vi "New Stainless Correction Pop Up.vi"(2 "New Feet\n of Stainless\n(Count)":i32) -> (0 "Feet of\nStainless to be\nUsed (Count)":i32)   [LabVIEW 2016]
doc: "This vi allows the clinician to input the starting flexion. It used in order to derive a flexion correction."
uses:
  Kpro Globals.vi
panel:
  out "Depth to Water Table":dbl=-5.0 format="%.2f"
  out "Original Feet\n of Stainless\n(Count)":i32
  in  "stop":bool
  in  "Increment Stainless":bool
  in  "Stainless OK As Is":bool
  in  "Correct Stainless":bool
  # "Please Choose \nto Correct, Increment, or to \nLeave Feet of Stainless as is"
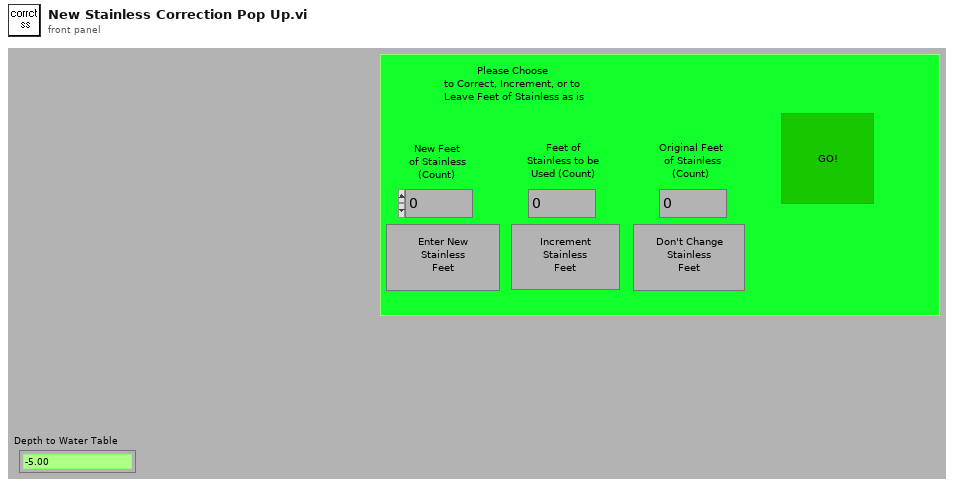
[diagram p1: front panel]
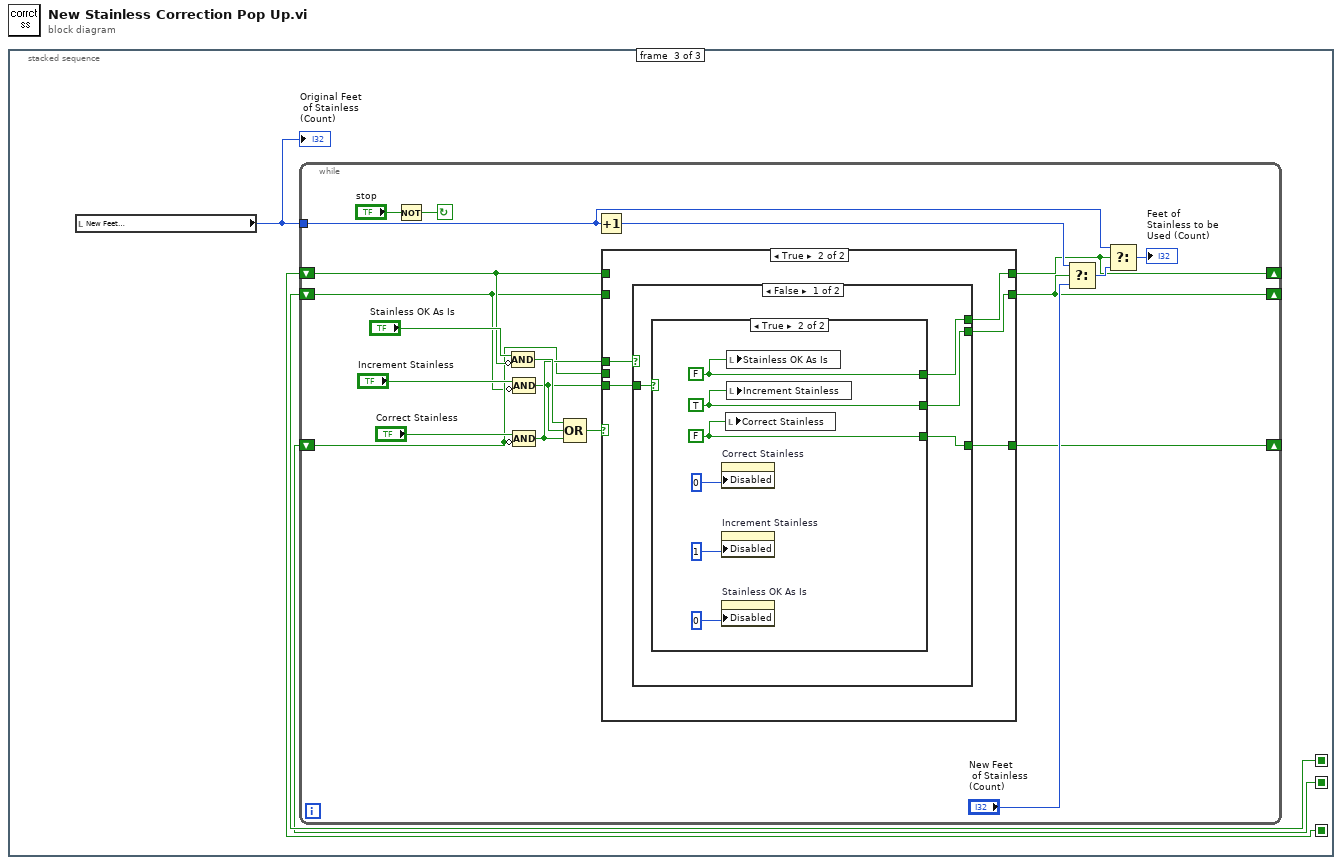
[diagram p0: block diagram]
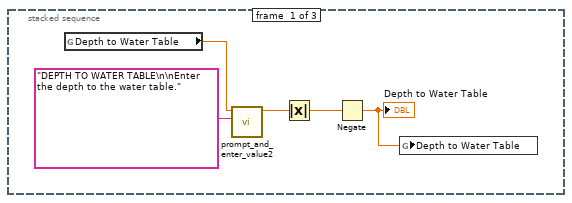
[diagram p2: hidden frame]
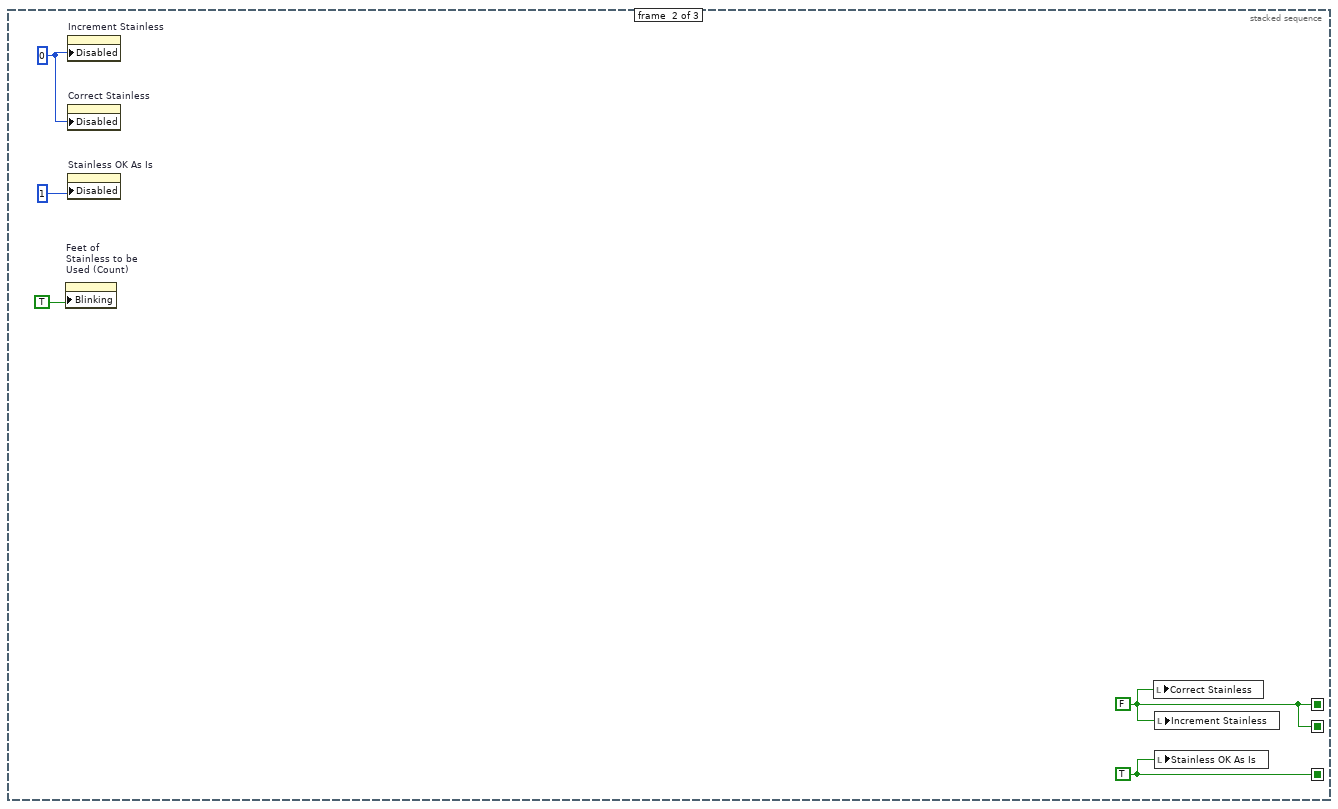
[diagram p3: hidden frame]
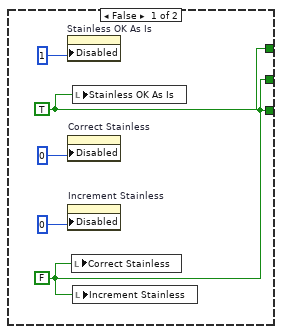
[diagram p5: hidden frame]
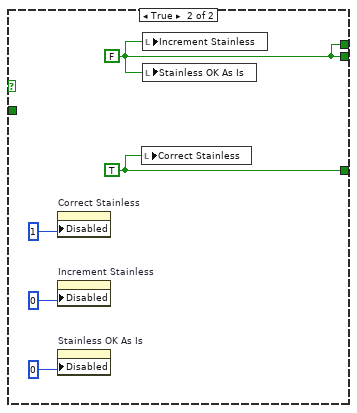
[diagram p6: hidden frame]
diagram:
  n1 = stacked-sequence {
    seq-local: [_ w9 _] -> [_ _ w12]
    seq-local: [_ w9 _] -> [_ _ w13]
    seq-local: [_ w10 _] -> [_ _ w14]
    frame #0 {
      n2 = global read "Kpro Globals.vi" "Depth to Water Table"() -> (w5:dbl)
      n3 = call "prompt_and_enter_value2.vi"("prompt_IN"="DEPTH TO WATER TABLE\n\nEnter the depth to the water table." ("prompt"), "Enter value"=w5) -> ("Numeric"=w1:dbl)  [unwired: 9 in]
      n4 = Absolute Value(x=w1) -> (abs(x)=w2:dbl)
      n5 = Negate(x=w2) -> (-x=w3:dbl)
      "Depth to Water Table" <- w3
      n6 = global write "Kpro Globals.vi" "Depth to Water Table"(w3) -> ()
    }
    frame #1 {
      w7 = 0
      w10 = TRUE
      w9 = FALSE
      n7 = property on="Feet of\nStainless to be\nUsed (Count)" class="DigNum (strict)"("Blinking"=TRUE) -> ()  [unwired: 2 in, 2 out]
      n8 = property on="Increment Stainless" class="Bool (strict)"("Disabled"=w7) -> ()  [unwired: 2 in, 2 out]
      n9 = property on="Correct Stainless" class="Bool (strict)"("Disabled"=w7) -> ()  [unwired: 2 in, 2 out]
      n10 = property on="Stainless OK As Is" class="Bool (strict)"("Disabled"=1) -> ()  [unwired: 2 in, 2 out]
      n11 = local write "Correct Stainless"(w9) -> ()
      n12 = local write "Increment Stainless"(w9) -> ()
      n13 = local write "Stainless OK As Is"(w10) -> ()
    }
    frame #2 {
      n14 = local read "New Feet\n of Stainless\n(Count)"() -> (w11:i32)
      "Original Feet\n of Stainless\n(Count)" <- w11
      n15 = while {
        tunnel: w11 -> [w16]
        shift-left: w12 -> [w18]
        shift-right: [w23] -> _
        shift-left: w13 -> [w17]
        shift-right: [w24] -> _
        shift-left: w14 -> [w19]
        shift-right: [w15] -> _
        stop <- w20 continue-if-true
        n16 = Not(x="stop") -> (.not. x?=w20:bool)
        n17 = Compound Arithmetic op=AND("Stainless OK As Is", invert w19) -> (w26:bool)
        n18 = Compound Arithmetic op=AND("Increment Stainless", invert w17) -> (w21:bool)
        n19 = Compound Arithmetic op=AND("Correct Stainless", invert w18) -> (w22:bool)
        n20 = Compound Arithmetic op=OR(w26, w21, w22) -> (w25:bool)
        n21 = Increment(x=w16) -> (x+1=w33:i32)
        n22 = case shown="True" w25 {
          tunnel: [w37 w40] -> w15
          tunnel: [w36 w39] -> w24
          tunnel: [w35 w41] -> w23
          tunnel: w22 -> [_ w42]
          tunnel: w21 -> [_ w38]
          tunnel: w19 -> [w37 _]
          tunnel: w18 -> [w35 _]
          tunnel: w17 -> [w36 _]
          frame False {
          }
          frame True {
            n23 = case shown="False" w42 {
              tunnel: [w43 w62] -> w41
              tunnel: [w45 w61] -> w40
              tunnel: [w44 w61] -> w39
              tunnel: w38 -> [w46 _]
              frame False {
                n24 = case shown="True" w46 {
                  tunnel: [w50 w55] -> w45
                  tunnel: [w51 w56] -> w44
                  tunnel: [w51 w57] -> w43
                  frame False {
                    w50 = TRUE
                    w51 = FALSE
                    n25 = property on="Stainless OK As Is" class="Bool (strict)"("Disabled"=1) -> ()  [unwired: 2 in, 2 out]
                    n26 = property on="Correct Stainless" class="Bool (strict)"("Disabled"=0) -> ()  [unwired: 2 in, 2 out]
                    n27 = property on="Increment Stainless" class="Bool (strict)"("Disabled"=0) -> ()  [unwired: 2 in, 2 out]
                    n28 = local write "Correct Stainless"(w51) -> ()
                    n29 = local write "Stainless OK As Is"(w50) -> ()
                    n30 = local write "Increment Stainless"(w51) -> ()
                  }
                  frame True {
                    w55 = FALSE
                    w56 = TRUE
                    w57 = FALSE
                    n31 = property on="Correct Stainless" class="Bool (strict)"("Disabled"=0) -> ()  [unwired: 2 in, 2 out]
                    n32 = property on="Increment Stainless" class="Bool (strict)"("Disabled"=1) -> ()  [unwired: 2 in, 2 out]
                    n33 = property on="Stainless OK As Is" class="Bool (strict)"("Disabled"=0) -> ()  [unwired: 2 in, 2 out]
                    n34 = local write "Correct Stainless"(w57) -> ()
                    n35 = local write "Stainless OK As Is"(w55) -> ()
                    n36 = local write "Increment Stainless"(w56) -> ()
                  }
                }
              }
              frame True {
                w61 = FALSE
                w62 = TRUE
                n37 = property on="Correct Stainless" class="Bool (strict)"("Disabled"=1) -> ()  [unwired: 2 in, 2 out]
                n38 = property on="Increment Stainless" class="Bool (strict)"("Disabled"=0) -> ()  [unwired: 2 in, 2 out]
                n39 = property on="Stainless OK As Is" class="Bool (strict)"("Disabled"=0) -> ()  [unwired: 2 in, 2 out]
                n40 = local write "Correct Stainless"(w62) -> ()
                n41 = local write "Increment Stainless"(w61) -> ()
                n42 = local write "Stainless OK As Is"(w61) -> ()
              }
            }
          }
        }
        n43 = Select(t=w33, s=w24, f="New Feet\n of Stainless\n(Count)") -> (s? t:f=w32:i32)
        n44 = Select(t=w16, s=w15, f=w32) -> (s? t:f=→"Feet of\nStainless to be\nUsed (Count)":i32)
      }
    }
  }
